vi "WD_SWB_Update_database.vi"(7 "計算用array":cluster{"條碼A":string, "條碼B":string}[](array[cluster])=[{"條碼A"="", "條碼B"="80540"}, {"條碼A"="7834", "條碼B"="80540"}, {"條碼A"="453", "條碼B"="453"}], 8 "error in (no error)":errorcluster, 9 "站點總數":i32=5, 10 "當前料數":i32=2, 11 "DBLink":string="Driver={ODBC Driver 17 for SQL Server};Server=localhost\\SQLEXPRESS;Database=ZDX201;UID=labview;PWD=Dsa@54137926") -> (0 "error out":errorcluster)   [LabVIEW 2019]
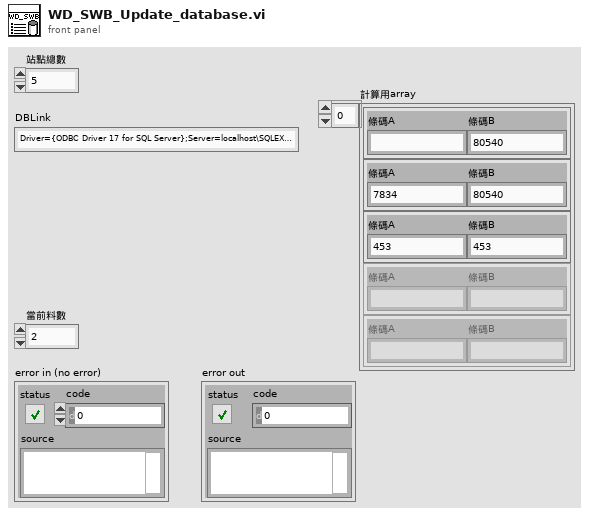
[diagram p1: front panel]
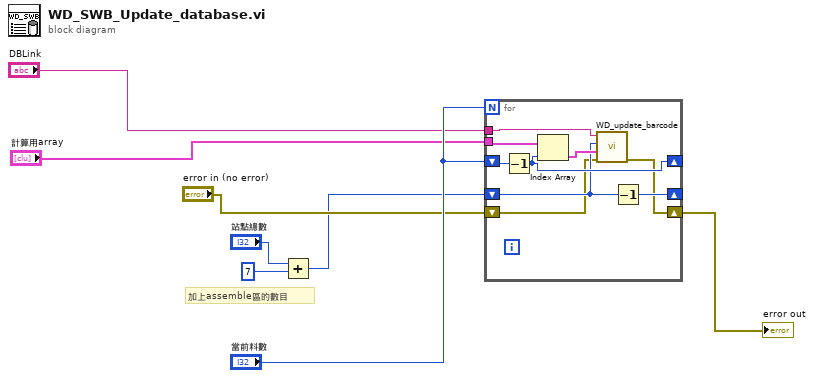
[diagram p0: block diagram]
diagram:
  # "加上assemble區的數目"
  n1 = Add(x="站點總數", y=7) -> (x+y=w1:i32)
  n2 = for {
    N: "當前料數" -> [_]
    shift-right: [w9] -> w5
    shift-left: "error in (no error)" -> [w10]
    tunnel: "計算用array" -> [w17]
    shift-right: [w13] -> _
    shift-left: "當前料數" -> [w16]
    tunnel: "DBLink" -> [w14]
    shift-right: [w12] -> _
    shift-left: w1 -> [w11]
    n3 = Decrement(x=w16) -> (x-1=w13:i32)
    n4 = Index Array(array=w17, index=w13) -> (element=w15:cluster{"條碼A":string, "條碼B":string})
    n5 = call "WD_update_barcode.vi"("error in (no error)"=w10, "Workplace data"=w15, "workplace_id"=w11, "DBlink"=w14) -> ("error out"=w9:errorcluster)  [unwired: 7 in]
    n6 = Decrement(x=w11) -> (x-1=w12:i32)
  }
  "error out" <- w5
